vi "Read_register _values_2.vi"(8 "error in":errorcluster, 11 "Register":T1(ring)) -> (0 "error out":errorcluster, 3 "Data":u16)   [LabVIEW 2018]
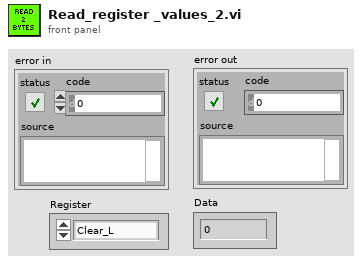
[diagram p1: front panel]
types:
  T1 = enum8{"Clear_L", "Clear_H", "Red_L", "Red_H", "Green_L", "Green_H", "Blue_L", "Blue_H"}
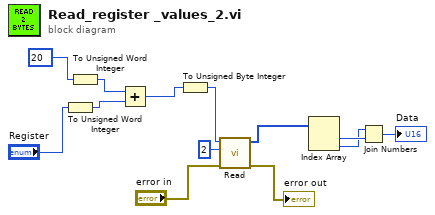
[diagram p0: block diagram]
diagram:
  n1 = To Unsigned Word Integer(number="Register") -> (unsigned 16bit integer=w2:u16)
  n2 = To Unsigned Word Integer(number=u8 20 ("Slave Address (7-bit)")) -> (unsigned 16bit integer=w3:u16)
  n3 = Add(x=w3, y=w2) -> (x+y=w12:u16)
  n4 = To Unsigned Byte Integer(number=w12) -> (unsigned 8bit integer=w11:u8)
  n5 = call "Read.vi"("error in"="error in", "Byte Count"=u32 2, "Byte to Write"=w11) -> ("error out"=→"error out":errorcluster, "Bytes Read"=w5:u8[])  [unwired: 7 in]
  n6 = Index Array(array=w5) -> (element #1=w8:u8, element #2=w7:u8)  [unwired: 2 in]
  n7 = Join Numbers(hi=w7, lo=w8) -> ((hi.lo)=→"Data":u16)
